vi "Convert-Baud-Rate.vi"(10 "FPGA Clock Rate (MHz)":u32=100, 11 "Baud Rate":u32(ring)=128000 items=["110"=110, "300"=300, "1200"=1200, "2400"=2400, "4800"=4800, "9600"=9600, "19200"=19200, "38400"=38400, "57600"=57600, "115200"=115200, "128000"=128000, "230400"=230400, "460800"=460800, "921600"=921600]) -> (0 "Two Bit":u32, 1 "One and Half Bit":u32, 2 "One Bit":u32, 3 "Half Bit":u32)   [LabVIEW 2017]
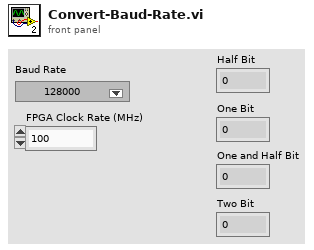
[diagram p1: front panel]
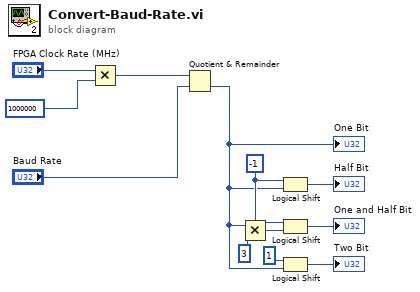
[diagram p0: block diagram]
diagram:
  w10 = i16 -1 ("y")
  n1 = Multiply(x="FPGA Clock Rate (MHz)", y=u32 1000000) -> (x*y=w3:u32)
  n2 = Quotient & Remainder(x=w3, y="Baud Rate") -> (floor(x/y)=w8:u32)  [unwired: 1 out]
  "One Bit" <- w8
  n3 = Multiply(x=w8, y=u32 3) -> (x*y=w12:u32)
  n4 = Logical Shift(y=w10, x=w8) -> (x << y=→"Half Bit":u32)
  n5 = Logical Shift(y=w10, x=w12) -> (x << y=→"One and Half Bit":u32)
  n6 = Logical Shift(y=i16 1, x=w8) -> (x << y=→"Two Bit":u32)
